vi "CRYReport Pic Out Log.vi"(6 "vi reference":refnum<vi>, 11 "sData":string) -> ()   [LabVIEW 2013]
uses:
  CRYWindow/SubVI/CRYMain Sub Window Global.vi
  CRYWindow/DataView/VIEW/CRYView Global.vi
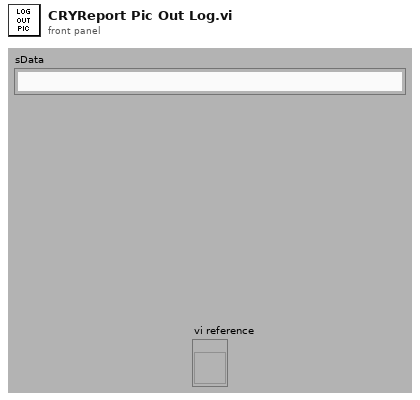
[diagram p1: front panel]
types:
  T1 = enum16{"open", "open or create", "create or replace", "create", "open (read only)"}
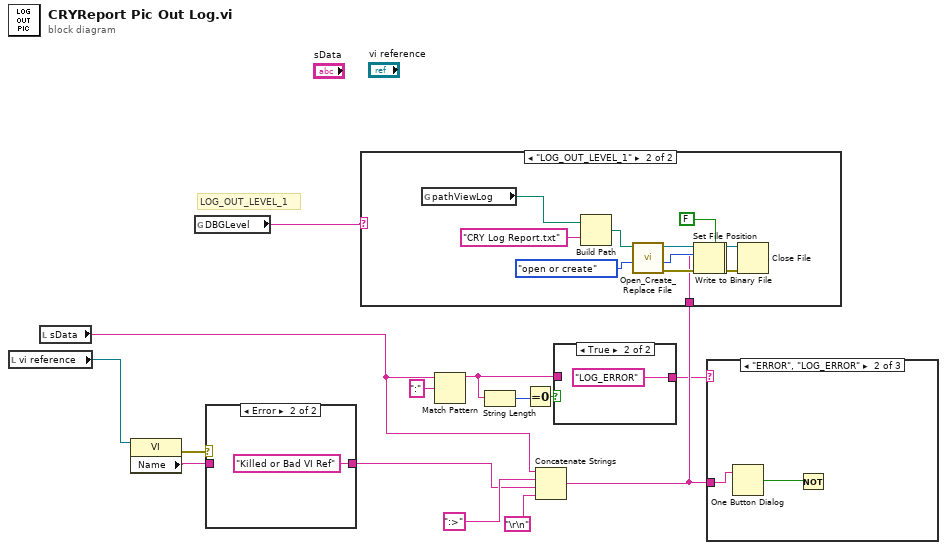
[diagram p0: block diagram]
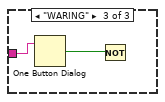
[diagram p6: hidden frame]
diagram:
  # "LOG_OUT_LEVEL_1"
  n1 = local read "vi reference"() -> (w14:refnum<vi>)
  n2 = local read "sData"() -> (w10:string)
  n3 = property class="VI"(reference=w14) -> (error out=w3:errorcluster, "Name"=w2:string)  [unwired: 1 in, 1 out]
  n4 = global read "CRYMain Sub Window Global.vi" "DBGLevel"() -> (w1:string)
  n5 = case shown="Error" w3 {
    tunnel: w2 -> [w15 _]
    tunnel: [w15 "Killed or Bad VI Ref" ("Name")] -> w9
    frame No Error {
    }
    frame Error {
    }
  }
  n6 = Match Pattern(string=w10, regular expression=":") -> (before substring=w5:string)  [unwired: 1 in, 3 out]
  n7 = String Length(string=w5) -> (length=w7:i32)
  n8 = Equal To 0?(x=w7) -> (x = 0?=w6:bool)
  n9 = Concatenate Strings(w10, ":>" ("string"), w9, "\r\n") -> (w8:string)
  n10 = case shown="\"LOG_OUT_LEVEL_1\"" w1 {
    tunnel: w8 -> [_ w18]
    frame Default {
    }
    frame "LOG_OUT_LEVEL_1" {
      n11 = global read "CRYView Global.vi" "pathViewLog"() -> (w17:path)
      n12 = Build Path(base path=w17, name or relative path="CRY Log Report.txt" ("name")) -> (appended path=w19:path)
      n13 = call <vilib>:"Open_Create_Replace File.vi"("function (open:0)"=T1."open or create", "file path"=w19) -> ("error out"=w27:errorcluster, "file size (bytes)"=w25:i32, "refnum"=w26:refnum<file>)  [unwired: 6 in, 1 out]
      n14 = Set File Position(offset (in bytes) (0)=w25, refnum=w26, error in=w27) -> (refnum out=w22:refnum<file>, error out=w21:errorcluster)  [unwired: 1 in]
      n15 = Write to Binary File(file (use dialog)=w22, data=w18, error in=w21, 5:FALSE ("prepend array or string size? (T)")) -> (refnum out=w23:refnum<file>, error out=w24:errorcluster)  [unwired: 2 in, 1 out]
      n16 = Close File(refnum=w23, error in=w24) -> ()  [unwired: 2 out]
    }
  }
  n17 = case shown="True" w6 {
    tunnel: [w30 "LOG_ERROR" ("sData")] -> w4
    tunnel: w5 -> [w30 _]
    frame False {
    }
    frame True {
    }
  }
  n18 = case shown="\"ERROR\", \"LOG_ERROR\"" w4 {
    tunnel: w8 -> [_ w32 w34]
    frame Default {
    }
    frame "ERROR", "LOG_ERROR" {
      n19 = One Button Dialog(message=w32) -> (true=w33:bool)  [unwired: 1 in]
      n20 = Not(x=w33) -> ()  [unwired: 1 out]
    }
    frame "WARING" {
      n21 = One Button Dialog(message=w34) -> (true=w35:bool)  [unwired: 1 in]
      n22 = Not(x=w35) -> ()  [unwired: 1 out]
    }
  }
